vi "General_2DGaussianfun.vi"(3 "output control":T1, 4 "data":variant, 5 "X":dbl[](array[numeric]), 6 "Coefficients":dbl[](array[numeric])) -> (0 "error out":errorcluster, 1 "f'(X,a)":dbl[][](array[numeric]), 2 "f(X,a)":dbl[](array[numeric]))   [LabVIEW 2014]
uses:
  <vilib>/gmath/NumericalOptimization/LM_output select.ctl
  <vilib>/gmath/NI_Gmath.lvlib
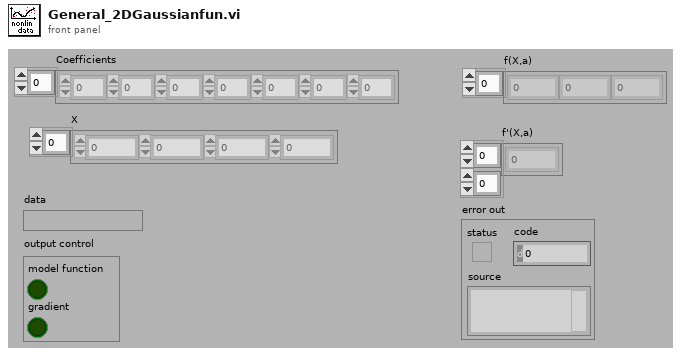
[diagram p1: front panel]
types:
  T1 = typedef "NI_Gmath.lvlib/LM_output select.ctl" = cluster{"model function":bool, "gradient":bool}
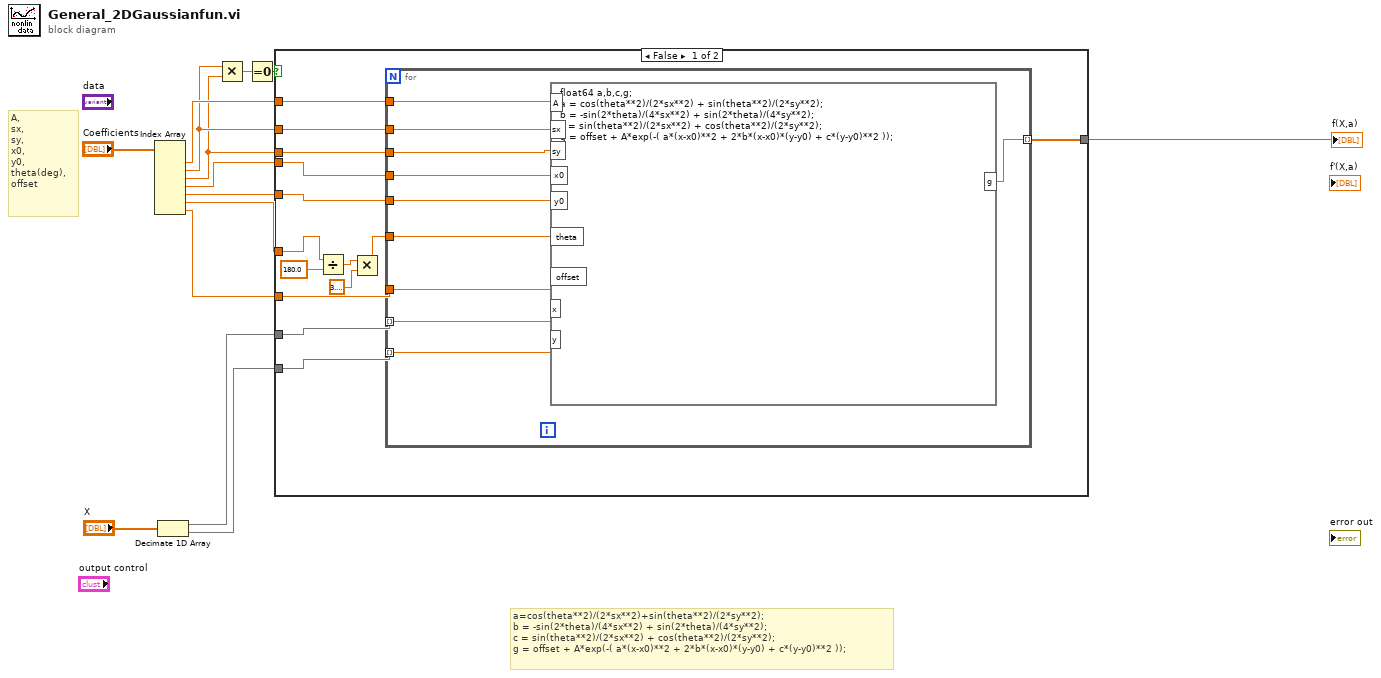
[diagram p0: block diagram]
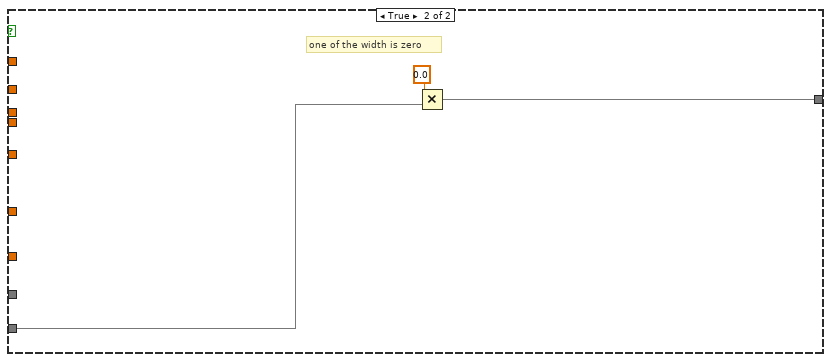
[diagram p2: hidden frame]
diagram:
  # "a=cos(theta**2)/(2*sx**2)+sin(theta**2)/(2*sy**2);\nb = -sin(2*theta)/(4*sx**2) + sin(2*theta)/(4*sy**2);\nc = sin(theta**2)/(2*sx**2) + cos(theta**2)/(2*sy**2);\ng = offset + A*exp(-( a*(x-x0)**2 + 2*b*(x-x0)*(y-y0) + c*(y-y0)**2 ));"
  # "A, \nsx, \nsy, \nx0, \ny0, \ntheta(deg), \noffset"
  n1 = Index Array(array="Coefficients") -> (element #1=w14:dbl, element #2=w3:dbl, element #3=w2:dbl, element #4=w11:dbl, element #5=w7:dbl, element #6=w4:dbl, element #7=w1:dbl)  [unwired: 7 in]
  n2 = Decimate 1D Array("X") -> (w13:dbl[], w12:dbl[])
  n3 = Multiply(x=w3, y=w2) -> (x*y=w10:dbl)
  n4 = Equal To 0?(x=w10) -> (x = 0?=w9:bool)
  n5 = case shown="False" w9 {
    tunnel: w14 -> [w28 _]
    tunnel: w13 -> [w22 _]
    tunnel: w12 -> [w21 w39]
    tunnel: w11 -> [w25 _]
    tunnel: [w20 w40] -> w5
    tunnel: w7 -> [w24 _]
    tunnel: w4 -> [w19 _]
    tunnel: w3 -> [w27 _]
    tunnel: w2 -> [w26 _]
    tunnel: w1 -> [w23 _]
    frame False {
      n6 = Divide(x=w19, y=180.0) -> (x/y=w17:dbl)
      n7 = Multiply(x=w17, y=3.141592653589793) -> (x*y=w15:dbl)
      n8 = for {
        tunnel: w28 -> [w38]
        tunnel: w27 -> [w37]
        tunnel: w26 -> [w36]
        tunnel: w25 -> [w35]
        tunnel: w24 -> [w34]
        tunnel: w15 -> [w33]
        tunnel: w23 -> [w32]
        tunnel: w22 -> [w31] mode=indexing
        tunnel: w21 -> [w30] mode=indexing
        tunnel: [w29] -> w20 mode=indexing
        n9 = formula code="float64 a,b,c,g;\na = cos(theta**2)/(2*sx**2) + sin(theta**2)/(2*sy**2);\nb = -sin(2*theta)/(4*sx**2) + sin(2*theta)/(4*sy**2);\nc = sin(theta**2)/(2*sx**2) + cos(theta**2)/(2*sy**2);\ng = offset + A*exp(-( a*(x-x0)**2 + 2*b*(x-x0)*(y-y0) + c*(y-y0)**2 ));"("A"=w38, "sx"=w37, "sy"=w36, "x0"=w35, "y0"=w34, "theta"=w33, "offset"=w32, "x"=w31, "y"=w30) -> ("g"=w29:dbl)
      }
    }
    frame True {
      # "one of the width is zero"
      n10 = Multiply(x=0.0, y=w39) -> (x*y=w40:dbl[])
    }
  }
  "f(X,a)" <- w5
